vi "Kill pixels.vi"(4 "Killing list":T1(array[cluster]) {"ChipID" format="%.0x"}, 5 "EQ folder path":string) -> (1 "ChipIDs to reprogram":u16[](array[numeric]) format="%04x")   [LabVIEW 2015, in "VIPM2.lvlib"]
uses:
  VIPM2.lvlib
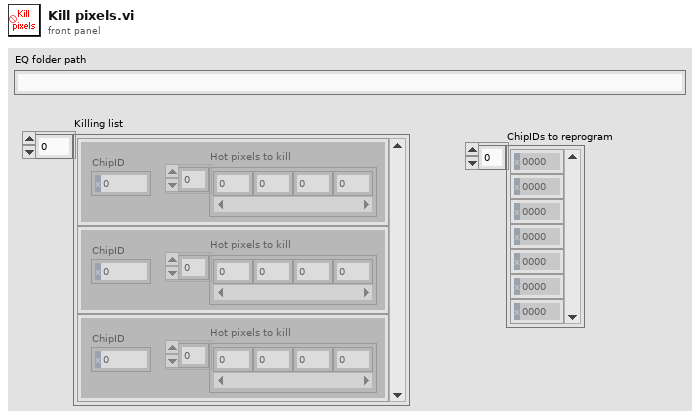
[diagram p1: front panel]
types:
  T1 = cluster{"ChipID":u16, "Hot pixels to kill":u8[]}[]
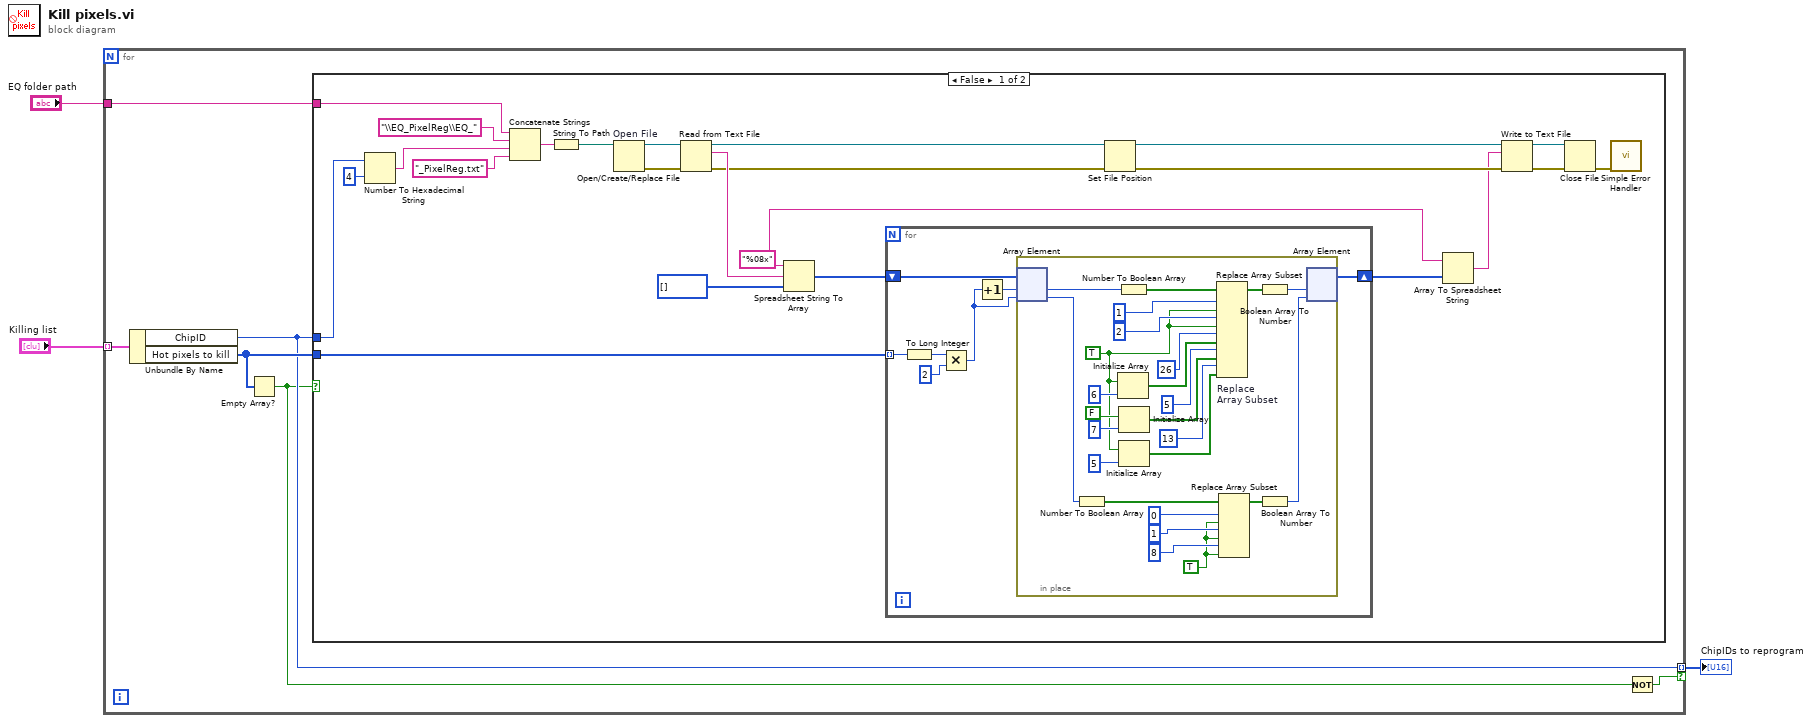
[diagram p0: block diagram]
diagram:
  n1 = for {
    tunnel: "EQ folder path" -> [w8]
    tunnel: "Killing list" -> [w9] mode=indexing
    tunnel: [w6] -> w1 mode=indexing if=w5
    n2 = Unbundle By Name(w9) -> ("ChipID"=w6:u16, "Hot pixels to kill"=w7:u8[])
    n3 = Empty Array?(array=w7) -> (empty?=w4:bool)
    n4 = case shown="False" w4 {
      tunnel: w8 -> [w30 _]
      tunnel: w6 -> [w29 _]
      tunnel: w7 -> [w21 _]
      frame False {
        w17 = "%08x" ("format string")
        n5 = Number To Hexadecimal String(1:i16 4 ("width (-)"), 2:w29) -> (0:w27:string)
        n6 = Concatenate Strings(w30, "\\EQ_PixelReg\\EQ_", w27, "_PixelReg.txt") -> (w31:string)
        n7 = String To Path(string=w31) -> (path=w26:path)
        n8 = Open/Create/Replace File "Open File"(file path (use dialog)=w26) -> (refnum out=w25:refnum<file>, error out=w24:errorcluster)  [unwired: 5 in, 1 out]
        n9 = Read from Text File(file (use dialog)=w25, error in=w24) -> (refnum out=w16:refnum<file>, text=w23:string, error out=w15:errorcluster)  [unwired: 2 in, 1 out]
        n10 = Spreadsheet String To Array(format string=w17, spreadsheet string=w23, array type (2D Dbl)=u32[] []) -> (array=w20:u32[])  [unwired: 1 in]
        n11 = for {
          tunnel: w21 -> [w39] mode=indexing
          shift-right: [w38] -> w18
          shift-left: w20 -> [w40]
          n12 = To Long Integer(number=w39) -> (32bit integer=w36:i32)
          n13 = Multiply(x=w36, y=2) -> (x*y=w34:i32)
          n14 = Increment(x=w34) -> (x+1=w37:i32)
          n15 = in-place "In Place Element Structure" {
            w49 = TRUE
            w47 = TRUE
            n16 = in-place-array #1(w40, w37, w34) -> (w44:u32, w43:u32)
            n17 = Number To Boolean Array(number=w43) -> (Boolean array=w54:bool[])
            n18 = Initialize Array(w47, 6 ("dimension size")) -> (w58:bool[])
            n19 = Number To Boolean Array(number=w44) -> (Boolean array=w65:bool[])
            n20 = Initialize Array(FALSE, 7 ("dimension size")) -> (w60:bool[])
            n21 = Initialize Array(w47, 5 ("dimension size")) -> (w45:bool[])
            n22 = Replace Array Subset "Replace \nArray Subset"(array=w65, new element #1=w47, index #1=1 ("index"), new element #2=w47, index #2=2 ("index"), new element #3=w58, index #3=26 ("index"), new element #4=w60, index #4=5 ("index"), new element #5=w45, index #5=13 ("index")) -> (w64:bool[])
            n23 = Replace Array Subset(array=w54, new element #1=w49, index #1=0 ("index"), new element #2=w49, index #2=1 ("index"), new element #3=w49, index #3=8 ("index")) -> (w53:bool[])
            n24 = Boolean Array To Number(Boolean array=w64) -> (number=w42:u32)
            n25 = Boolean Array To Number(Boolean array=w53) -> (number=w41:u32)
            n26 = in-place-array #1(w42, w41) -> (w38:u32[])  [unwired: 2 out]
          }
        }
        n27 = Set File Position(refnum=w16, error in=w15) -> (refnum out=w14:refnum<file>, error out=w13:errorcluster)  [unwired: 2 in]
        n28 = Array To Spreadsheet String(array=w18, 3:w17) -> (spreadsheet string=w12:string)  [unwired: 1 in]
        n29 = Write to Text File(file (use dialog)=w14, text=w12, error in=w13) -> (refnum out=w11:refnum<file>, error out=w10:errorcluster)  [unwired: 1 in, 1 out]
        n30 = Close File(refnum=w11, error in=w10) -> (error out=w22:errorcluster)  [unwired: 1 out]
        n31 = call <vilib>:"Simple Error Handler.vi"("error in (no error)"=w22) -> ()  [unwired: 4 in, 5 out]
      }
      frame True {
      }
    }
    n32 = Not(x=w4) -> (.not. x?=w5:bool)
  }
  "ChipIDs to reprogram" <- w1
